vi "CC Script Parser Test Program.vi"(8 "error in (no error)":errorcluster) -> (0 "error out":errorcluster)   [LabVIEW 2020]
uses:
  typedefs/CC cluster RA and DEC.ctl
panel:
  out "RA and DEC":T1
  out "DEC String":string
  out "RA String":string
  out "Declination":T2 {"Arc Sec" format="%0#2_6g"}
  out "Right Ascension":T3
  in  "RA and DEC String":cluster{"RA":string, "DEC":string}={"RA"="HH:MM:SS.nnn", "DEC"="DEG:arcmin:arcsec.nn"} caption="RA and DEC"
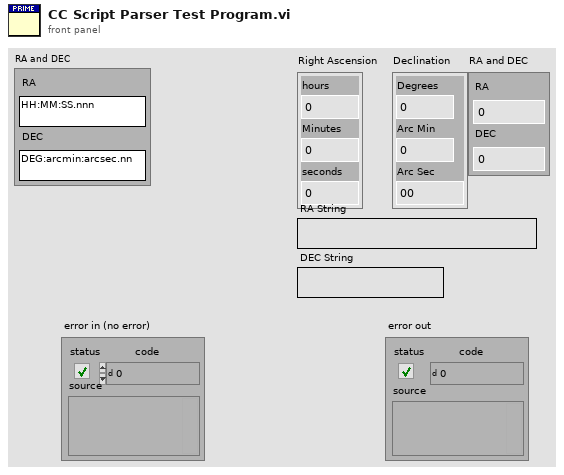
[diagram p1: front panel]
types:
  T1 = typedef "CC cluster RA and DEC.ctl" = cluster{"RA":dbl, "DEC":dbl}
  T2 = cluster{"Degrees":dbl, "Arc Min":dbl, "Arc Sec":dbl}
  T3 = cluster{"hours":dbl, "Minutes":dbl, "seconds":dbl}
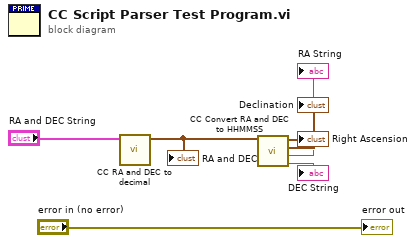
[diagram p0: block diagram]
diagram:
  n1 = call "CC RA and DEC to decimal.vi"("RA and DEC String"="RA and DEC String") -> ("RA and DEC"=w6:T1)  [unwired: 9 in, 1 out]
  "RA and DEC" <- w6
  n2 = call "CC Convert RA and DEC to HHMMSS.vi"("RA and DEC"=w6) -> ("DEC String"=→"DEC String":string, "RA String"=→"RA String":string, "Declination"=→"Declination":T2, "Right Ascension"=→"Right Ascension":T3)  [unwired: 7 in]
  "error out" <- "error in (no error)"
